vi "Parse Measurement(hot garbage).vi"(6 "Measurement Line":string) -> (13 "Voltage":dbl, 14 "Measure String Array":string[](array[string]), 15 "Frequency":dbl, 16 "Capacitance":dbl format="%#_10f", 17 "Loss":dbl format="%#_10f", 18 "Units":i32(ring) items=["", "nanosiemens", "dissipation factor", "kilohms", "gigohms", "loss vector (jpF)"], 19 "Loss Greater Than":bool)   [LabVIEW 2017, in "Andeen-Hagerling 2700.lvlib"]
doc: "This VI parses a text line of measurement results from the bridge. Measurement results are dependent on the labelling parameter of Format and the Field parameters. Boolean inputs are provided to represent these parameters. These only need to be set if the the Format or Field are not set as in the Default Instrument Setup VI."
uses:
  <userlib>/_probes/default/AH2700/Andeen-Hagerling 2700/Andeen-Hagerling 2700.lvlib
panel:
  # "Measurement Results"
  # "Format Parameter"
  # "Field Parameters"
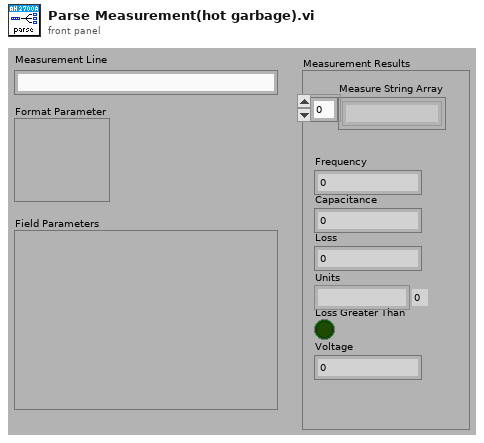
[diagram p1: front panel]
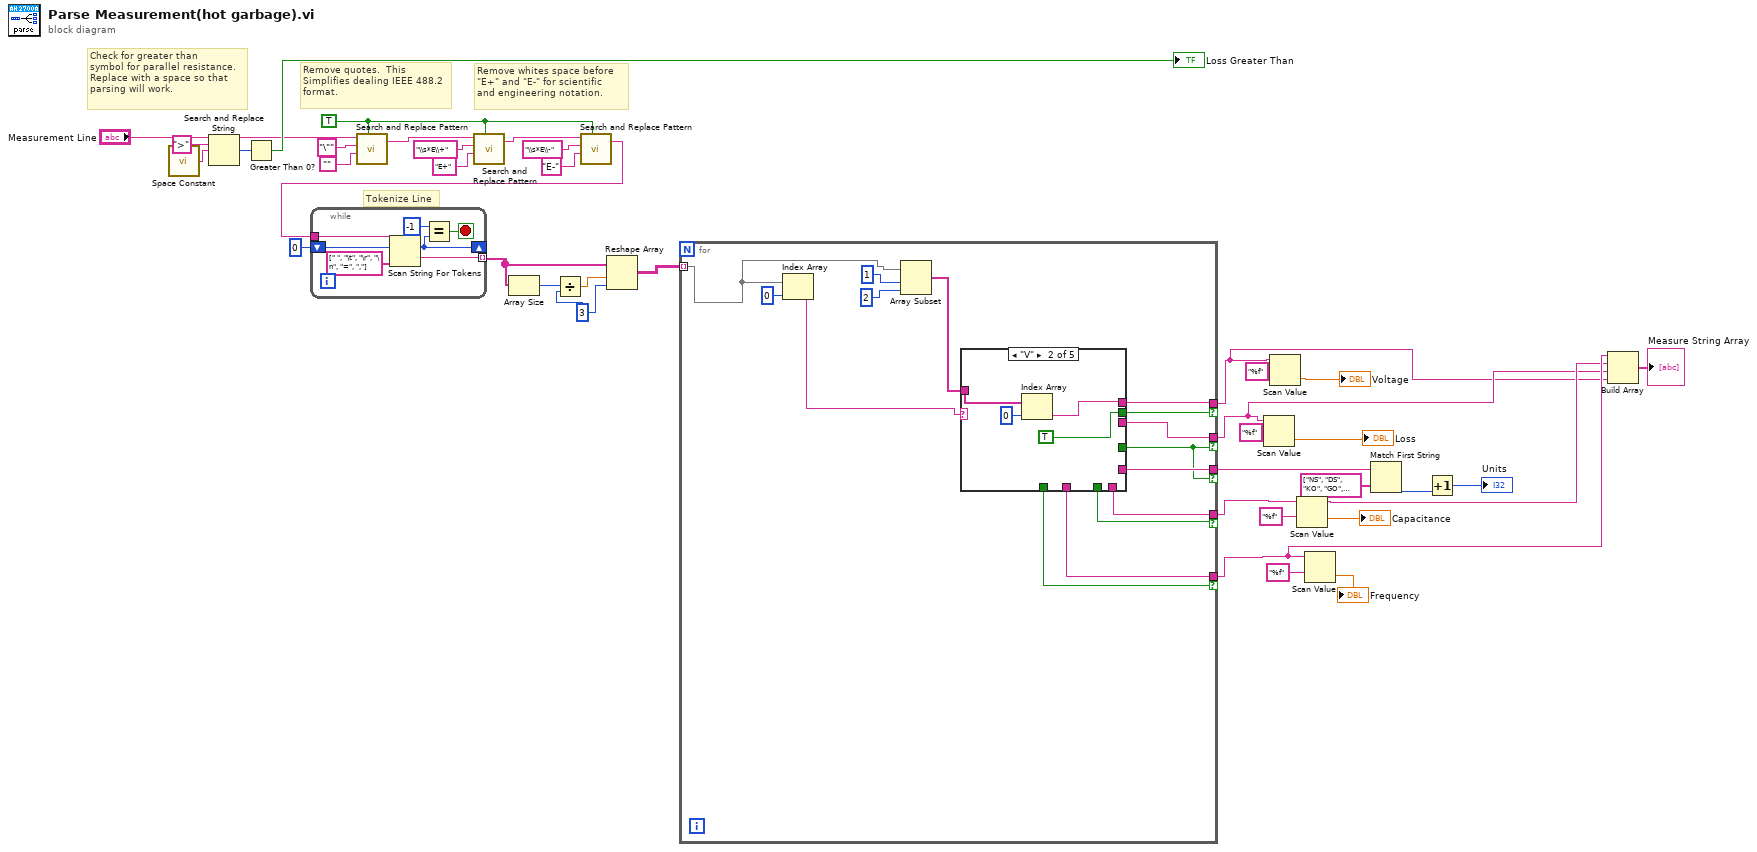
[diagram p0: block diagram]
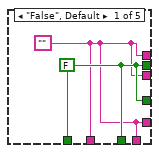
[diagram p2: hidden frame]
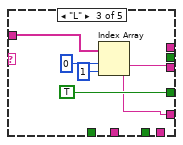
[diagram p3: hidden frame]
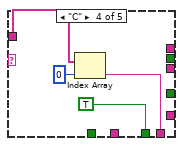
[diagram p4: hidden frame]
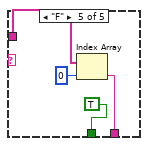
[diagram p5: hidden frame]
diagram:
  w19 = 3 ("dimension size")
  w25 = TRUE ("replace all? (F)")
  # "Remove quotes.  This\nSimplifies dealing IEEE 488.2\nformat."
  # "Remove whites space before\n\"E+\" and \"E-\" for scientific\nand engineering notation."
  # "Tokenize Line"
  # "Check for greater than\nsymbol for parallel resistance.\nReplace with a space so that\nparsing will work."
  n1 = call <vilib>:"Space Constant.vi"() -> ("String"=w37:string)
  n2 = Search and Replace String(input string="Measurement Line", search string=">", replace string=w37) -> (result string=w24:string, number of replacements=w38:i32)  [unwired: 5 in, 2 out]
  n3 = Greater Than 0?(x=w38) -> (x > 0?=→"Loss Greater Than":bool)
  n4 = call <vilib>:"Search and Replace Pattern.vi"("string"=w24, "regular expression (\"\")"="\"" ("regular expression (\"\")"), "replace string (\"\")"="", "replace all? (F)"=w25) -> ("result string"=w28:string)  [unwired: 1 in, 1 out]
  n5 = call <vilib>:"Search and Replace Pattern.vi"("string"=w28, "regular expression (\"\")"="\\s*E\\+" ("regular expression (\"\")"), "replace string (\"\")"="E+" ("replace string (\"\")"), "replace all? (F)"=w25) -> ("result string"=w29:string)  [unwired: 1 in, 1 out]
  n6 = call <vilib>:"Search and Replace Pattern.vi"("string"=w29, "regular expression (\"\")"="\\s*E\\-" ("regular expression (\"\")"), "replace string (\"\")"="E-" ("replace string (\"\")"), "replace all? (F)"=w25) -> ("result string"=w23:string)  [unwired: 1 in, 1 out]
  n7 = while {
    tunnel: [w45] -> w21 mode=indexing
    tunnel: w23 -> [w44]
    shift-right: [w42] -> _
    shift-left: 0 ("token index") -> [w43]
    stop <- w46 stop-if-true
    n8 = Scan String For Tokens(6:string[] [" ", "\t", "\r", "\n", "=", ","] ("delimiters (\\s,\\t,\\r,\\n)"), 8:w43, 9:w44) -> (1:w45:string, 2:w42:i32)  [unwired: 3 in, 2 out]
    n9 = Equal?(x=-1 ("y"), y=w42) -> (x = y?=w46:bool)
  }
  n10 = Array Size(array=w21) -> (size(s)=w22:i32)
  n11 = Divide(x=w22, y=w19) -> (x/y=w20:dbl)
  n12 = Reshape Array(w21, w20, w19) -> (w18:string[][])
  n13 = for {
    tunnel: w18 -> [w60] mode=indexing
    tunnel: [w55] -> w1 if=w50
    tunnel: [w54] -> w2 if=w47
    tunnel: [w53] -> w3 if=w48
    tunnel: [w52] -> w4 if=w49
    tunnel: [w51] -> w6 if=w47
    n14 = Index Array(array=w60, index=0) -> (element=w57:string)
    n15 = Array Subset(array=w60, index=1, length=2 ("index")) -> (w56:string[])
    n16 = case shown="\"V\"" w57 {
      tunnel: w56 -> [_ w66 w72 w75 w79]
      tunnel: [w62 w65 _ _ _] -> w55
      tunnel: [w62 _ w71 _ _] -> w54
      tunnel: [w62 _ _ w76 _] -> w53
      tunnel: [w62 _ _ _ w80] -> w52
      tunnel: [w62 _ w68 _ _] -> w51
      tunnel: [w63 TRUE _ _ _] -> w50
      tunnel: [w63 _ TRUE _ _] -> w47
      tunnel: [w63 _ _ TRUE _] -> w48
      tunnel: [w63 _ _ _ TRUE] -> w49
      frame "False", Default {
        w62 = ""
        w63 = FALSE
      }
      frame "V" {
        n17 = Index Array(array=w66, index=0) -> (element=w65:string)
      }
      frame "L" {
        n18 = Index Array(array=w72, index #1=0 ("index"), index #2=1 ("index")) -> (element #1=w71:string, element #2=w68:string)
      }
      frame "C" {
        n19 = Index Array(array=w75, index=0) -> (element=w76:string)
      }
      frame "F" {
        n20 = Index Array(array=w79, index=0) -> (element=w80:string)
      }
    }
  }
  n21 = Scan Value(string=w2, format string="%f") -> (value=→"Loss":dbl)  [unwired: 1 in, 1 out]
  n22 = Scan Value(string=w1, format string="%f") -> (value=→"Voltage":dbl)  [unwired: 1 in, 1 out]
  n23 = Scan Value(string=w3, format string="%f") -> (value=→"Capacitance":dbl)  [unwired: 1 in, 1 out]
  n24 = Scan Value(string=w4, format string="%f") -> (value=→"Frequency":dbl)  [unwired: 1 in, 1 out]
  n25 = Match First String(2:string[] ["NS", "DS", "KO", "GO", "JP"] ("string array"), 3:w6) -> (0:w16:i32)  [unwired: 1 out]
  n26 = Increment(x=w16) -> (x+1=→"Units":i32)
  n27 = Build Array(w4, w3, w2, w1) -> (→"Measure String Array":string[])
